vi "HDT.vi"(0 "System no.":i32=1 min=1 max=4 step=1, 2 "DeviceID":i32[](array[numeric]), 5 "error in":errorcluster, 6 "DeviceAxis":i32[](array[numeric]), 10 "TableID":i32[](array[numeric])) -> (14 "Controller error":bool, 19 "error out":errorcluster)   [LabVIEW 2026]
doc: "This VI assigns a lookup table to the given axis of the given Human Interface Device (HID), waits 100 ms and queries ERR?. See controller user manual for details. Controller error is TRUE if selected system reports error code unequal to 0. \n\nC-867: Lookup tables are assigned in volatile memory only (RAM). Use WPA to save the current assignment to non-volatile memory. See controller user manual for details. \n\nC-884, E-871, E-872, E-873: Lookup tables are assigned in volatile memory only (RAM). Use WPA to save the current assignment to non-volatile memory. See controller user manual for details."
panel:
  # "This vi assigns a lookup table to the given axis of the given Human Interface Device (HID), waits 100 ms and queries ERR?."
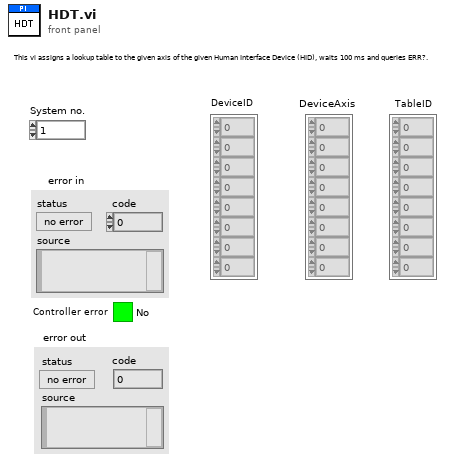
[diagram p1: front panel]
types:
  T1 = enum16{"Disable error check", "Force error check", "Use global settings"}
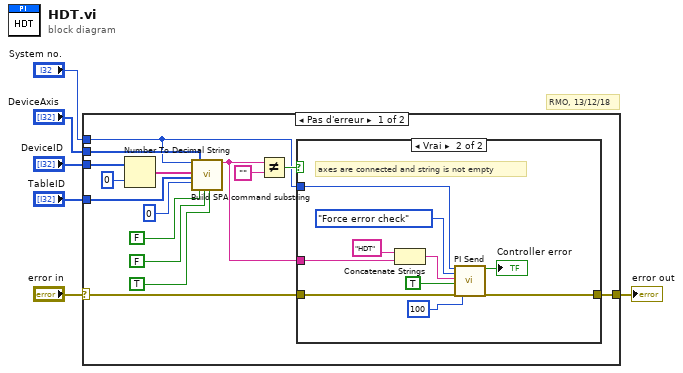
[diagram p0: block diagram]
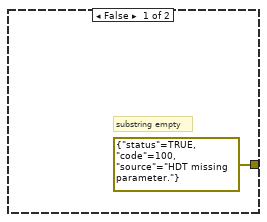
[diagram p2: hidden frame]
diagram:
  # "RMO, 13/12/18"
  n1 = case shown="Pas d'erreur" "error in" {
    selector: "error in" -> [w7 w33]
    tunnel: [w21 w33] -> w6
    tunnel: "System no." -> [w16 _]
    tunnel: "DeviceID" -> [w12 _]
    tunnel: "DeviceAxis" -> [w18 _]
    tunnel: "TableID" -> [w8 _]
    frame No Error {
      n2 = Number To Decimal String(number=w12, width (-)=i16 0) -> (decimal integer string=w10:string[])
      n3 = call "Build SPA command substring.vi"("System no."=w16, "Axes to set"=w10, "Parameter values"=w8, "No. of digits"=i16 0, "Parameter number"=w18, "Parameter no. format \n(Decimal: FALSE)"=FALSE ("Parameter no. format \n(Decimal: FALSE)"), "Parameter format \n(Num.: FALSE)"=FALSE ("Parameter format \n(Num.: FALSE)"), "With space?"=TRUE) -> ("SPA command substring"=w19:string)  [unwired: 2 in, 9 out]
      n4 = Not Equal?(x=w19, y="") -> (x != y?=w17:bool)
      n5 = case shown="Vrai" w17 {
        tunnel: w19 -> [_ w31]
        tunnel: [errorcluster {"status"=TRUE, "code"=100, "source"="HDT missing parameter."} ("error out") w25] -> w21
        tunnel: w7 -> [_ w28]
        tunnel: w16 -> [_ w27]
        frame False {
          # "substring empty"
        }
        frame True {
          # "axes are connected and string is not empty"
          n6 = Concatenate Strings("HDT", w31) -> (w29:string)
          n7 = call "PI Send.vi"("System no."=w27, "Error check settings"=T1."Force error check", "String to send"=w29, "Attach termination char.?"=TRUE ("Attach Linefeed?"), "error in"=w28, "Delay before error check (ms)"=u32 100 ("milliseconds to wait")) -> ("Controller error"=→"Controller error":bool, "error out"=w25:errorcluster)  [unwired: 12 out]
        }
      }
    }
    frame Error {
    }
  }
  "error out" <- w6
